vi "EOL Digital Output Tasks.vi"(8 "error in":errorcluster, 11 "path":path=path "C:/Labview Code/System/Digital Output Channel Configuration") -> (0 "error out":errorcluster, 3 "DO Tasks":refnum<k21>[](array[refnum]))   [LabVIEW 2018]
uses:
  <vilib>/Utility/file.llb/Read From Spreadsheet File (string).vi
  <vilib>/DAQmx/create/channels.llb/DAQmx Create Channel (DO-Digital Output).vi
panel:
  out "配置信息":string[][](array[string])
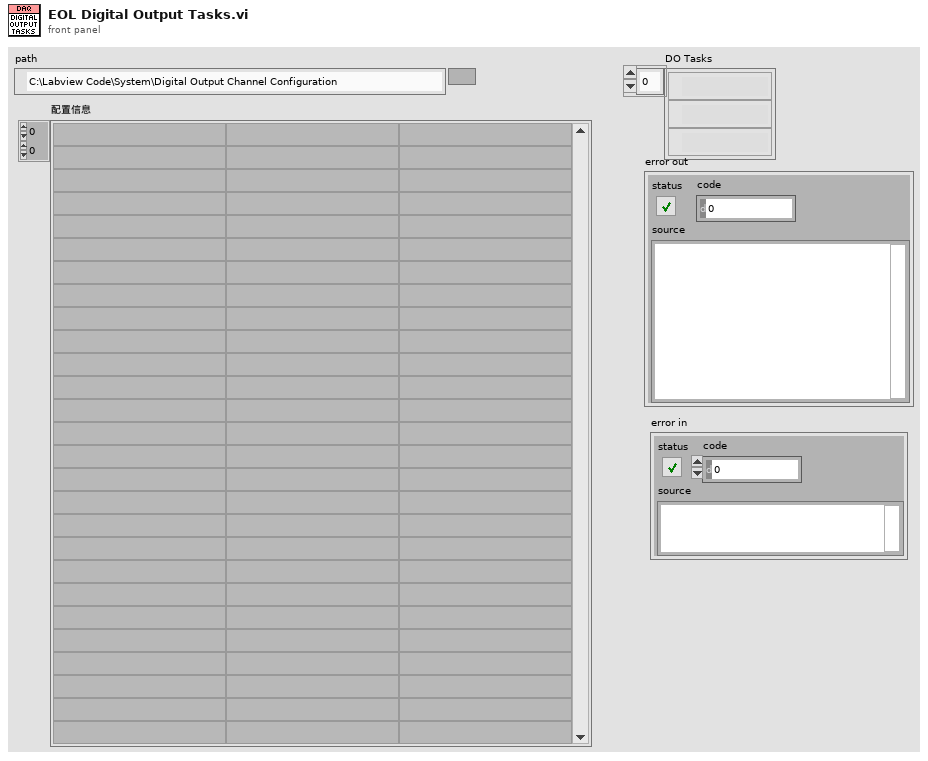
[diagram p1: front panel]
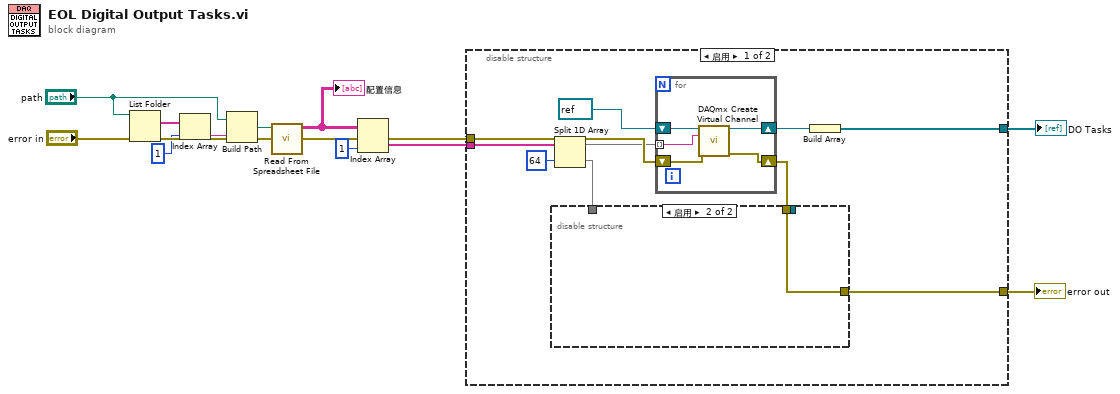
[diagram p0: block diagram]
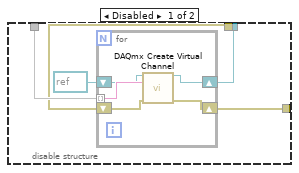
[diagram p2: hidden frame]
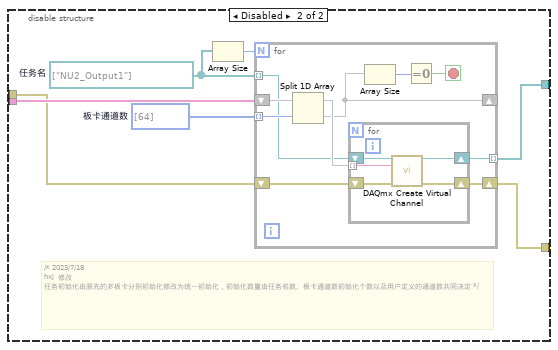
[diagram p3: hidden frame]
diagram:
  n1 = List Folder(path="path", error in="error in") -> (filenames=w9:string[], error out=w5:errorcluster)  [unwired: 2 in, 2 out]
  n2 = Index Array(array=w9, index=1 ("索引")) -> (element=w8:string)
  n3 = Build Path(base path="path", name or relative path=w8) -> (appended path=w6:path)
  n4 = call-poly <vilib>:"Read From Spreadsheet File.vi"("file path (dialog if empty)"=w6) -> ("all rows"=w12:string[][])  [unwired: 6 in, 4 out]
  "配置信息" <- w12
  n5 = Index Array(array=w12, index (col)=1 ("disabled index (col)")) -> (element=w1:string[])  [unwired: 1 in]
  n6 = disable-structure shown="启用" {
    disable-tunnel: w1 -> [w22 w45]
    disable-tunnel: [w21 w41] -> w10
    disable-tunnel: w5 -> [w20 w40]
    disable-tunnel: [w14 w39] -> w2
    frame Enabled {
      n7 = Split 1D Array(array=w22, index=64) -> (first subarray=w18:string[], second subarray=w17:string[])
      n8 = for {
        tunnel: w18 -> [w36] mode=indexing
        shift-right: [w38] -> w16
        shift-left: refnum<k21> refnum ("task out") -> [w37]
        shift-right: [w34] -> w15
        shift-left: w20 -> [w35]
        n9 = call-poly <vilib>:"DAQmx Create Virtual Channel.vi"("task in"=w37, "lines"=w36, "error in"=w35) -> ("task out"=w38:refnum<k21>, "error out"=w34:errorcluster)  [unwired: 11 in]
      }
      n10 = disable-structure shown="启用" {
        disable-tunnel: w17 -> [w26 _]
        disable-tunnel: [w25 _] -> _
        disable-tunnel: w15 -> [w24 w33]
        disable-tunnel: [w23 w33] -> w14
        frame Disabled {
          n11 = for {
            tunnel: w26 -> [w31] mode=indexing
            shift-right: [w32] -> w25
            shift-left: refnum<k21> refnum ("task out") -> [w30]
            shift-right: [w28] -> w23
            shift-left: w24 -> [w29]
            n12 = call-poly <vilib>:"DAQmx Create Virtual Channel.vi"("task in"=w30, "lines"=w31, "error in"=w29) -> ("task out"=w32:refnum<k21>, "error out"=w28:errorcluster)  [unwired: 11 in]
          }
        }
        frame Enabled {
        }
      }
      n13 = Build Array(w16) -> (w21:refnum<k21>[])
    }
    frame Disabled {
      w43 = i32[] [64]  # 板卡通道数
      w42 = refnum<k21>[] ["NU2_Output1"]  # 任务名
      # "/* 2023/7/18\nhxj  修改\n任务初始化由原先的多板卡分别初始化修改为统一初始化，初始化数量由任务名数、板卡通道数初始化个数以及用户定义的通道数共同决定 */"
      n14 = Array Size(array=w42) -> (size(s)=w44:i32)
      n15 = for {
        N: w44 -> [_]
        tunnel: w43 -> [w54] mode=indexing
        tunnel: w42 -> [w52] mode=indexing
        shift-right: [w51] -> _
        shift-left: w45 -> [w55]
        tunnel: [w48] -> w41 mode=indexing
        shift-right: [w46] -> w39
        shift-left: w40 -> [w47]
        stop <- w49 stop-if-true
        n16 = Split 1D Array(array=w55, index=w54) -> (first subarray=w53:string[], second subarray=w51:string[])
        n17 = for {
          tunnel: w53 -> [w58] mode=indexing
          shift-right: [w60] -> w48
          shift-left: w52 -> [w59]
          shift-right: [w56] -> w46
          shift-left: w47 -> [w57]
          n18 = call-poly <vilib>:"DAQmx Create Virtual Channel.vi"("task in"=w59, "lines"=w58, "error in"=w57) -> ("task out"=w60:refnum<k21>, "error out"=w56:errorcluster)  [unwired: 11 in]
        }
        n19 = Array Size(array=w51) -> (size(s)=w50:i32)
        n20 = Equal To 0?(x=w50) -> (x = 0?=w49:bool)
      }
    }
  }
  "DO Tasks" <- w10
  "error out" <- w2
